vi "From JSON.vi"(7 "LVClass Serializer":refnum<class "JSONtext LVClass Serializer.lvclass">, 8 "error in (no error)":errorcluster, 10 "<JSON>":string, 11 "Fake JSON Serializable in":refnum<class "Fake JSON Serializable.lvclass">) -> (0 "error out":errorcluster, 3 "Fake JSON Serializable out":refnum<class "Fake JSON Serializable.lvclass">)   [LabVIEW 2017, in "JSON Serializable Binder Tests.lvlib" / "Fake JSON Serializable.lvclass"]
doc: "Reads data from a JSON string."
uses:
  Fake JSON Serializable.lvclass
  <vilib>/JDP Science/JSONtext/LVClass Serializer/JSONtext LVClass Serializer.lvclass
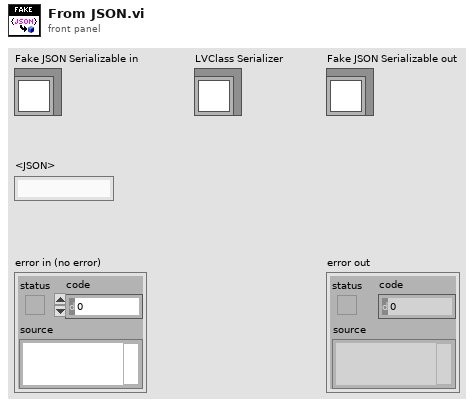
[diagram p1: front panel]
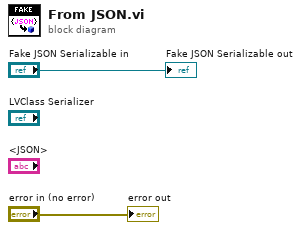
[diagram p0: block diagram]
diagram:
  "error out" <- "error in (no error)"
  "Fake JSON Serializable out" <- "Fake JSON Serializable in"
